vi "MGCC_PVFcst_main.vi"() -> ()   [LabVIEW 2016]
doc: "-----------------------------------------------------------------------------------------------------------------------\nCopyright <2019> <The University of Tennessee at Knoxville and the University of Tennessee Research Foundation>\nThis software is released under BSD-3 \nhttps://opensource.org/licenses/BSD-3-Clause \nAdditional license options available at https://utrf.tennessee.edu/industry/sample-agreements/\n-----------------------------------------------------------------------------------------------------------------------\n\n\nThis VI implements a PV forecasting algorithm using ARMA regression. The measurements from the PV local controller are taken every 15 minutes, and are stored using shared variables. Weather information is assumed to be available, and is transmitted through communication. The VI distinguishes between sunny and overcast days, but more detailed classification of cloud cover can be achieved using the same approach (case structure). The VI calls Sub-VI \"MGCC_PVFcst_PF.vi\" to train and generate forecasts for the next 24-hour period. If an alternative timing source is available, the timers in this VI can be replaced for free control of the triggering of this VI."
uses:
  Sub-VIs/f_MGCC_PVFcst_ActualPV.vi
  Finite State Machine/Sub-VIs/MGCC_FntStaMach_gobal.vi
  Finite State Machine/Sub-VIs/MGCC_FntStaMach_PV_Mode.vi
  Communication/Global communication.vi
  Communication/Global communication output.vi
  <vilib>/Utility/error.llb/Error Cluster From Error Code.vi
  <vilib>/ErrorRing/Error Ring.xnode
  <vilib>/Analysis/NI_AALBase.lvlib
  Lib/MGCC_PVFcst_dataIO.lvlib
panel:
  out "f_MGCC_PVFcst_HistoricalPV_Overcast":dbl[](graph)
  out "Forecast_overcast":dbl[](graph)
  out "f_MGCC_PVFcst_HistoricalPV_Sunny":dbl[](graph)
  out "Forecast_sunny":dbl[](graph)
  out "error1":errorcluster
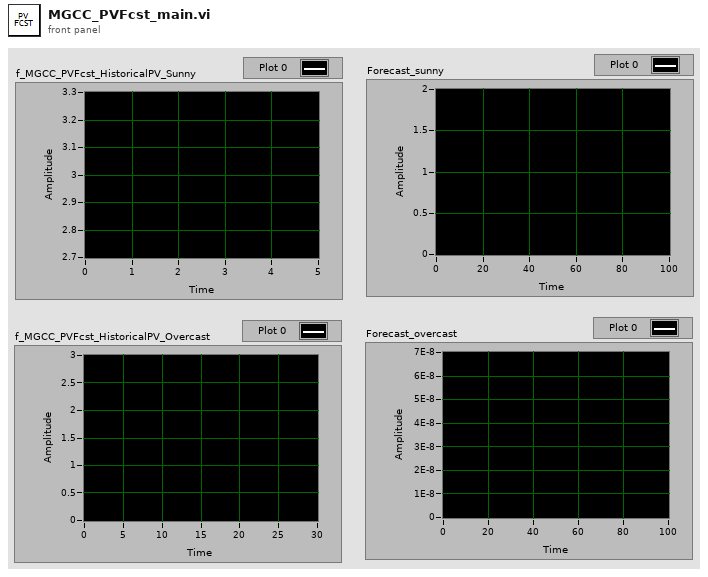
[diagram p1: front panel]
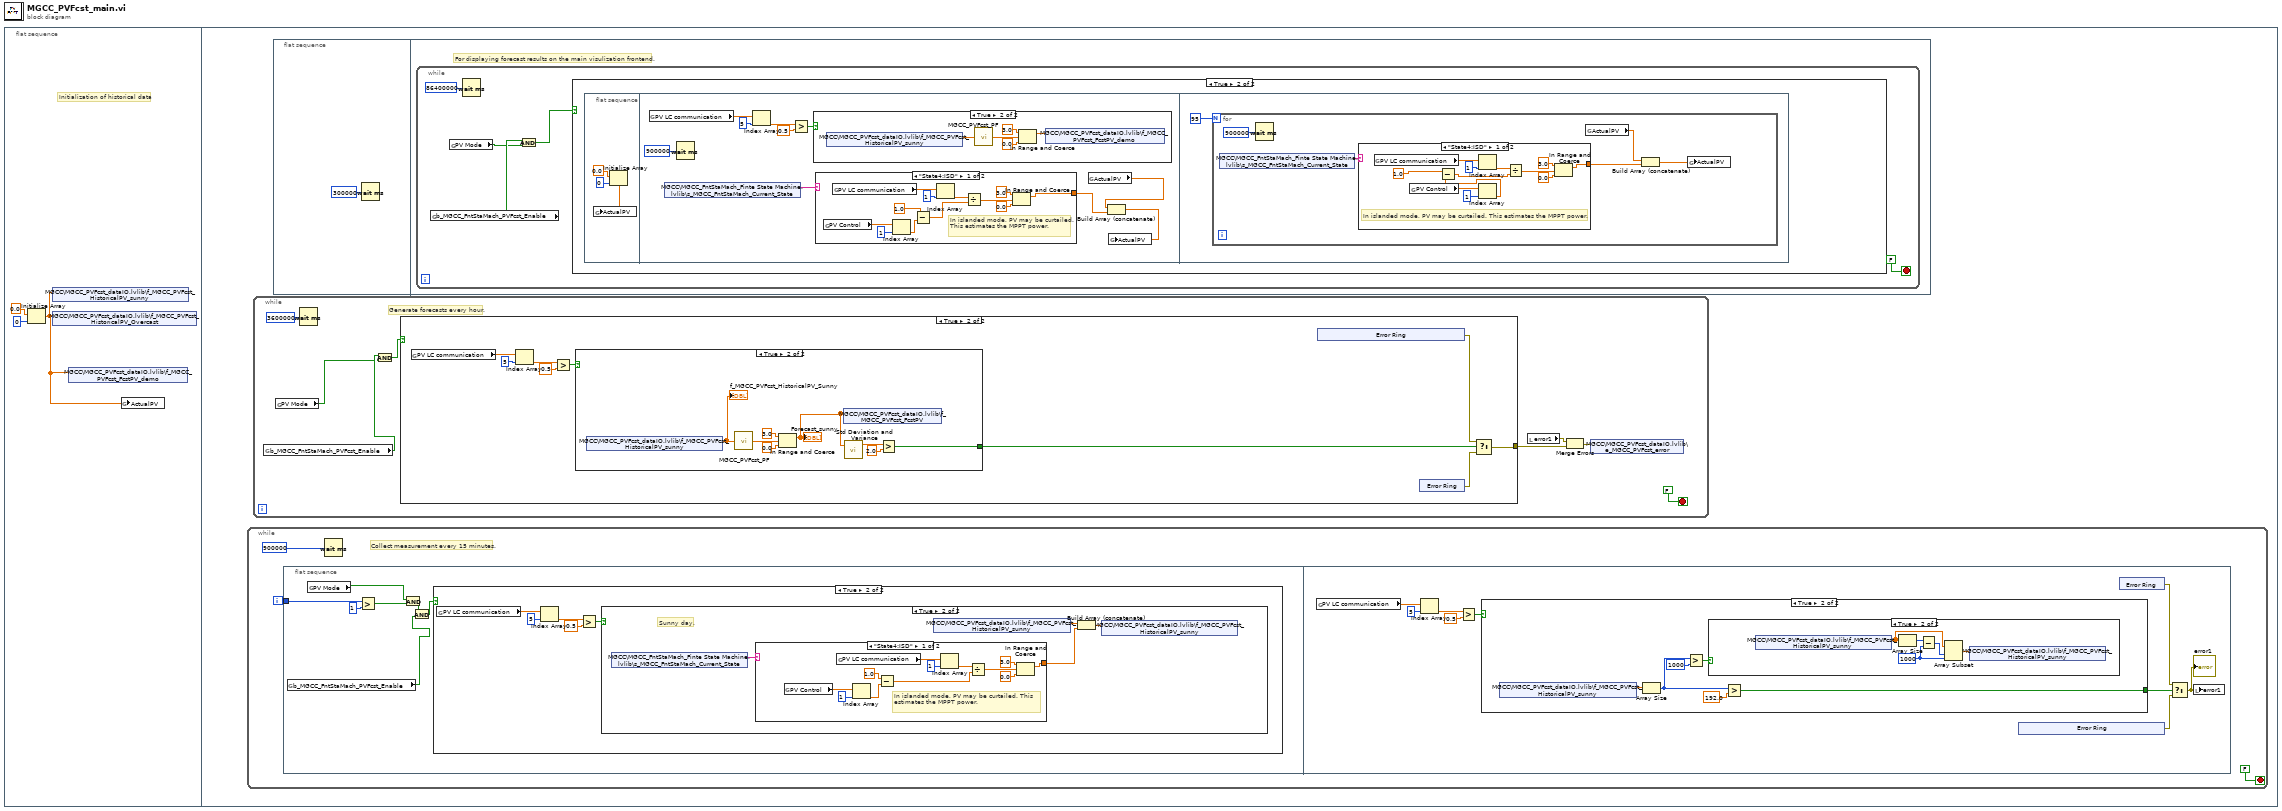
[diagram p0: block diagram]
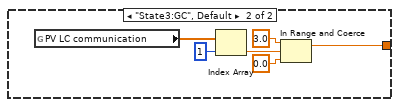
[diagram p3: hidden frame]
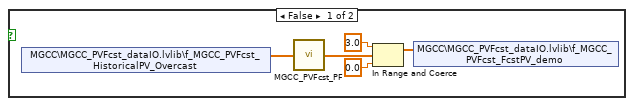
[diagram p4: hidden frame]
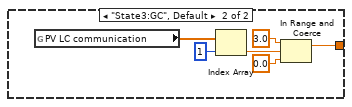
[diagram p5: hidden frame]
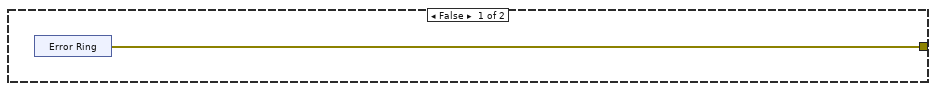
[diagram p6: hidden frame]
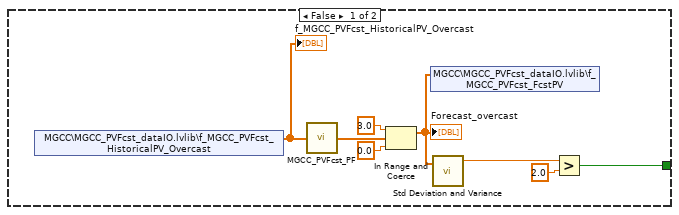
[diagram p7: hidden frame]
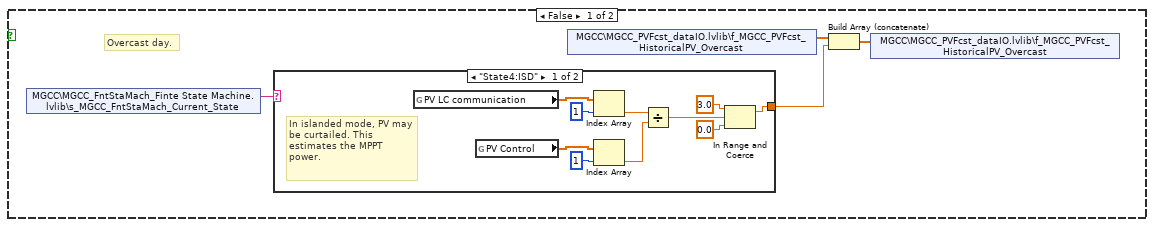
[diagram p9: hidden frame]
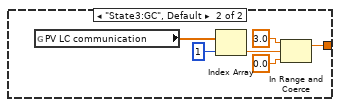
[diagram p10: hidden frame]
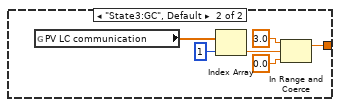
[diagram p11: hidden frame]
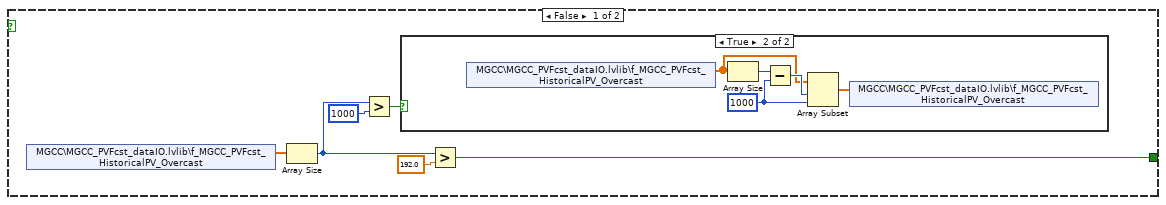
[diagram p12: hidden frame]
diagram:
  n1 = flat-sequence {
    frame #0 {
      # "Initialization of historical data"
      n2 = Initialize Array(0.0 ("element"), 0 ("dimension size")) -> (w1:dbl[])
      n3 = shared-variable "MGCC\\MGCC_PVFcst_dataIO.lvlib\\f_MGCC_PVFcst_HistoricalPV_sunny"(w1) -> ()  [unwired: 1 in, 1 out]
      n4 = shared-variable "MGCC\\MGCC_PVFcst_dataIO.lvlib\\f_MGCC_PVFcst_HistoricalPV_Overcast"(w1) -> ()  [unwired: 1 in, 1 out]
      n5 = shared-variable "MGCC\\MGCC_PVFcst_dataIO.lvlib\\f_MGCC_PVFcst_FcstPV_demo"(w1) -> ()  [unwired: 1 in, 1 out]
      n6 = global write "f_MGCC_PVFcst_ActualPV.vi" "ActualPV"(w1) -> ()
    }
    frame #1 {
      n7 = while {
        i -> [w116]
        stop <- FALSE stop-if-true
        # "Collect measurement every 15 minutes."
        n8 = flat-sequence {
          tunnel: w116 -> [w123]
          frame #0 {
            n9 = global read "MGCC_FntStaMach_gobal.vi" "b_MGCC_FntStaMach_PVFcst_Enable"() -> (w120:bool)
            n10 = global read "MGCC_FntStaMach_PV_Mode.vi" "PV Mode"() -> (w119:bool)
            n11 = Greater?(x=w123, y=1) -> (0:w124:bool)
            n12 = And(x=w119, y=w124) -> (x .and. y?=w122:bool)
            n13 = And(x=w122, y=w120) -> (x .and. y?=w121:bool)
            n14 = case shown="True" w121 {
              frame False {
              }
              frame True {
                n15 = global read "Global communication.vi" "PV LC communication"() -> (w130:dbl[])
                n16 = Index Array(array=w130, index=5) -> (element=w128:dbl)
                n17 = Greater?(x=w128, y=0.5) -> (0:w126:bool)
                n18 = case shown="True" w126 {
                  frame False {
                    # "Overcast day."
                    n19 = shared-variable "MGCC\\MGCC_FntStaMach_Finte State Machine.lvlib\\s_MGCC_FntStaMach_Current_State"() -> (w131:string)  [unwired: 1 in, 1 out]
                    n20 = case shown="\"State4:ISD\"" w131 {
                      tunnel: [w135 w148] -> w132
                      frame "State4:ISD" {
                        # "In islanded mode, PV may be curtailed. This estimates the MPPT power."
                        n21 = global read "Global communication.vi" "PV LC communication"() -> (w142:dbl[])
                        n22 = global read "Global communication output.vi" "PV Control"() -> (w139:dbl[])
                        n23 = Index Array(array=w142, index=1) -> (element=w136:dbl)
                        n24 = Index Array(array=w139, index=1) -> (element=w138:dbl)
                        n25 = Divide(x=w136, y=w138) -> (x/y=w137:dbl)
                        n26 = In Range and Coerce(upper limit=3.0, x=w137, lower limit=0.0) -> (coerced(x)=w135:dbl)  [unwired: 1 out]
                      }
                      frame "State3:GC", Default {
                        n27 = global read "Global communication.vi" "PV LC communication"() -> (w147:dbl[])
                        n28 = Index Array(array=w147, index=1) -> (element=w145:dbl)
                        n29 = In Range and Coerce(upper limit=3.0, x=w145, lower limit=0.0) -> (coerced(x)=w148:dbl)  [unwired: 1 out]
                      }
                    }
                    n30 = shared-variable "MGCC\\MGCC_PVFcst_dataIO.lvlib\\f_MGCC_PVFcst_HistoricalPV_Overcast"() -> (w134:dbl[])  [unwired: 1 in, 1 out]
                    n31 = Build Array (concatenate)(w134, w132) -> (w133:dbl[])
                    n32 = shared-variable "MGCC\\MGCC_PVFcst_dataIO.lvlib\\f_MGCC_PVFcst_HistoricalPV_Overcast"(w133) -> ()  [unwired: 1 in, 1 out]
                  }
                  frame True {
                    # "Sunny day."
                    n33 = shared-variable "MGCC\\MGCC_FntStaMach_Finte State Machine.lvlib\\s_MGCC_FntStaMach_Current_State"() -> (w152:string)  [unwired: 1 in, 1 out]
                    n34 = case shown="\"State4:ISD\"" w152 {
                      tunnel: [w158 w170] -> w151
                      frame "State4:ISD" {
                        # "In islanded mode, PV may be curtailed. This estimates the MPPT power."
                        n35 = global read "Global communication output.vi" "PV Control"() -> (w161:dbl[])
                        n36 = global read "Global communication.vi" "PV LC communication"() -> (w164:dbl[])
                        n37 = Index Array(array=w161, index=1) -> (element=w157:dbl)
                        n38 = Subtract(x=1.0, y=w157) -> (x-y=w155:dbl)
                        n39 = Index Array(array=w164, index=1) -> (element=w159:dbl)
                        n40 = Divide(x=w159, y=w155) -> (x/y=w160:dbl)
                        n41 = In Range and Coerce(upper limit=3.0, x=w160, lower limit=0.0) -> (coerced(x)=w158:dbl)  [unwired: 1 out]
                      }
                      frame "State3:GC", Default {
                        n42 = global read "Global communication.vi" "PV LC communication"() -> (w169:dbl[])
                        n43 = Index Array(array=w169, index=1) -> (element=w167:dbl)
                        n44 = In Range and Coerce(upper limit=3.0, x=w167, lower limit=0.0) -> (coerced(x)=w170:dbl)  [unwired: 1 out]
                      }
                    }
                    n45 = shared-variable "MGCC\\MGCC_PVFcst_dataIO.lvlib\\f_MGCC_PVFcst_HistoricalPV_sunny"() -> (w154:dbl[])  [unwired: 1 in, 1 out]
                    n46 = Build Array (concatenate)(w154, w151) -> (w153:dbl[])
                    n47 = shared-variable "MGCC\\MGCC_PVFcst_dataIO.lvlib\\f_MGCC_PVFcst_HistoricalPV_sunny"(w153) -> ()  [unwired: 1 in, 1 out]
                  }
                }
              }
            }
          }
          frame #1 {
            n48 = global read "Global communication.vi" "PV LC communication"() -> (w177:dbl[])
            n49 = Index Array(array=w177, index=5) -> (element=w175:dbl)
            n50 = Greater?(x=w175, y=0.5) -> (0:w173:bool)
            n51 = case shown="True" w173 {
              tunnel: [w183 w193] -> w179
              frame False {
                n52 = shared-variable "MGCC\\MGCC_PVFcst_dataIO.lvlib\\f_MGCC_PVFcst_HistoricalPV_Overcast"() -> (w184:dbl[])  [unwired: 1 in, 1 out]
                n53 = Array Size(array=w184) -> (size(s)=w187:i32)
                n54 = Greater?(x=w187, y=1000) -> (0:w182:bool)
                n55 = case shown="True" w182 {
                  frame False {
                  }
                  frame True {
                    w192 = 1000 ("y")
                    n56 = shared-variable "MGCC\\MGCC_PVFcst_dataIO.lvlib\\f_MGCC_PVFcst_HistoricalPV_Overcast"() -> (w188:dbl[])  [unwired: 1 in, 1 out]
                    n57 = Array Size(array=w188) -> (size(s)=w189:i32)
                    n58 = Subtract(x=w189, y=w192) -> (x-y=w190:i32)
                    n59 = Array Subset(array=w188, index=w190, length=w192) -> (w191:dbl[])
                    n60 = shared-variable "MGCC\\MGCC_PVFcst_dataIO.lvlib\\f_MGCC_PVFcst_HistoricalPV_Overcast"(w191) -> ()  [unwired: 1 in, 1 out]
                  }
                }
                n61 = Greater?(x=w187, y=192.0) -> (0:w183:bool)
              }
              frame True {
                n62 = shared-variable "MGCC\\MGCC_PVFcst_dataIO.lvlib\\f_MGCC_PVFcst_HistoricalPV_sunny"() -> (w198:dbl[])  [unwired: 1 in, 1 out]
                n63 = Array Size(array=w198) -> (size(s)=w194:i32)
                n64 = Greater?(x=w194, y=1000) -> (0:w196:bool)
                n65 = case shown="True" w196 {
                  frame False {
                  }
                  frame True {
                    w199 = 1000 ("y")
                    n66 = shared-variable "MGCC\\MGCC_PVFcst_dataIO.lvlib\\f_MGCC_PVFcst_HistoricalPV_sunny"() -> (w203:dbl[])  [unwired: 1 in, 1 out]
                    n67 = Array Size(array=w203) -> (size(s)=w202:i32)
                    n68 = Subtract(x=w202, y=w199) -> (x-y=w201:i32)
                    n69 = Array Subset(array=w203, index=w201, length=w199) -> (w200:dbl[])
                    n70 = shared-variable "MGCC\\MGCC_PVFcst_dataIO.lvlib\\f_MGCC_PVFcst_HistoricalPV_sunny"(w200) -> ()  [unwired: 1 in, 1 out]
                  }
                }
                n71 = Greater?(x=w194, y=192.0) -> (0:w193:bool)
              }
            }
            n72 = xnode "Error Ring"() -> ("error out"=w180:errorcluster)
            n73 = xnode "Error Ring"() -> ("error out"=w181:errorcluster)
            n74 = Select(t=w181, s=w179, f=w180) -> (s? t:f=w178:errorcluster)
            "error1" <- w178
            n75 = local write "error1"(w178) -> ()
          }
        }
        n76 = Wait (ms)(milliseconds to wait=u32 900000) -> ()  [unwired: 1 out]
      }
      n77 = while {
        stop <- FALSE stop-if-true
        # "Generate forecasts every hour."
        n78 = global read "MGCC_FntStaMach_gobal.vi" "b_MGCC_FntStaMach_PVFcst_Enable"() -> (w76:bool)
        n79 = global read "MGCC_FntStaMach_PV_Mode.vi" "PV Mode"() -> (w75:bool)
        n80 = Wait (ms)(milliseconds to wait=u32 3600000) -> ()  [unwired: 1 out]
        n81 = And(x=w76, y=w75) -> (x .and. y?=w77:bool)
        n82 = case shown="True" w77 {
          tunnel: [w83 w90] -> w80
          frame False {
            n83 = xnode "Error Ring"() -> ("error out"=w83:errorcluster)
          }
          frame True {
            n84 = global read "Global communication.vi" "PV LC communication"() -> (w89:dbl[])
            n85 = Index Array(array=w89, index=5) -> (element=w87:dbl)
            n86 = Greater?(x=w87, y=0.5) -> (0:w85:bool)
            n87 = case shown="True" w85 {
              tunnel: [w94 w102] -> w91
              frame False {
                n88 = shared-variable "MGCC\\MGCC_PVFcst_dataIO.lvlib\\f_MGCC_PVFcst_HistoricalPV_Overcast"() -> (w95:dbl[])  [unwired: 1 in, 1 out]
                "f_MGCC_PVFcst_HistoricalPV_Overcast" <- w95
                n89 = call "MGCC_PVFcst_PF.vi"("InputTimeSeries"=w95) -> ("predicted series"=w98:dbl[])
                n90 = In Range and Coerce(upper limit=3.0, x=w98, lower limit=0.0) -> (coerced(x)=w101:dbl[])  [unwired: 1 out]
                "Forecast_overcast" <- w101
                n91 = shared-variable "MGCC\\MGCC_PVFcst_dataIO.lvlib\\f_MGCC_PVFcst_FcstPV"(w101) -> ()  [unwired: 1 in, 1 out]
                n92 = call <vilib>:"Std Deviation and Variance.vi"("X"=w101) -> ("mean"=w100:dbl)  [unwired: 1 in, 2 out]
                n93 = Greater?(x=w100, y=2.0) -> (0:w94:bool)
              }
              frame True {
                n94 = shared-variable "MGCC\\MGCC_PVFcst_dataIO.lvlib\\f_MGCC_PVFcst_HistoricalPV_sunny"() -> (w109:dbl[])  [unwired: 1 in, 1 out]
                "f_MGCC_PVFcst_HistoricalPV_Sunny" <- w109
                n95 = call "MGCC_PVFcst_PF.vi"("InputTimeSeries"=w109) -> ("predicted series"=w106:dbl[])
                n96 = In Range and Coerce(upper limit=3.0, x=w106, lower limit=0.0) -> (coerced(x)=w103:dbl[])  [unwired: 1 out]
                "Forecast_sunny" <- w103
                n97 = shared-variable "MGCC\\MGCC_PVFcst_dataIO.lvlib\\f_MGCC_PVFcst_FcstPV"(w103) -> ()  [unwired: 1 in, 1 out]
                n98 = call <vilib>:"Std Deviation and Variance.vi"("X"=w103) -> ("mean"=w104:dbl)  [unwired: 1 in, 2 out]
                n99 = Greater?(x=w104, y=2.0) -> (0:w102:bool)
              }
            }
            n100 = xnode "Error Ring"() -> ("error out"=w93:errorcluster)
            n101 = xnode "Error Ring"() -> ("error out"=w92:errorcluster)
            n102 = Select(t=w93, s=w91, f=w92) -> (s? t:f=w90:errorcluster)
          }
        }
        n103 = local read "error1"() -> (w78:errorcluster)
        n104 = Merge Errors(w78, w80) -> (w79:errorcluster)
        n105 = shared-variable "MGCC\\MGCC_PVFcst_dataIO.lvlib\\e_MGCC_PVFcst_error"(w79) -> ()  [unwired: 1 in, 1 out]
      }
      n106 = flat-sequence {
        frame #0 {
          n107 = Wait (ms)(milliseconds to wait=u32 300000) -> ()  [unwired: 1 out]
        }
        frame #1 {
          # "For displaying forecast results on the main visulization frontend."
          n108 = while {
            stop <- FALSE stop-if-true
            n109 = global read "MGCC_FntStaMach_gobal.vi" "b_MGCC_FntStaMach_PVFcst_Enable"() -> (w6:bool)
            n110 = global read "MGCC_FntStaMach_PV_Mode.vi" "PV Mode"() -> (w5:bool)
            n111 = Wait (ms)(milliseconds to wait=u32 86400000) -> ()  [unwired: 1 out]
            n112 = And(x=w6, y=w5) -> (x .and. y?=w7:bool)
            n113 = case shown="True" w7 {
              frame False {
              }
              frame True {
                n114 = flat-sequence {
                  frame #0 {
                    n115 = Initialize Array(0.0 ("element"), 0 ("dimension size")) -> (w12:dbl[])
                    n116 = global write "f_MGCC_PVFcst_ActualPV.vi" "ActualPV"(w12) -> ()
                  }
                  frame #1 {
                    n117 = global read "Global communication.vi" "PV LC communication"() -> (w22:dbl[])
                    n118 = shared-variable "MGCC\\MGCC_FntStaMach_Finte State Machine.lvlib\\s_MGCC_FntStaMach_Current_State"() -> (w17:string)  [unwired: 1 in, 1 out]
                    n119 = Wait (ms)(milliseconds to wait=u32 900000) -> ()  [unwired: 1 out]
                    n120 = Index Array(array=w22, index=5) -> (element=w20:dbl)
                    n121 = Greater?(x=w20, y=0.5) -> (0:w18:bool)
                    n122 = case shown="True" w18 {
                      frame False {
                        n123 = shared-variable "MGCC\\MGCC_PVFcst_dataIO.lvlib\\f_MGCC_PVFcst_HistoricalPV_Overcast"() -> (w41:dbl[])  [unwired: 1 in, 1 out]
                        n124 = call "MGCC_PVFcst_PF.vi"("InputTimeSeries"=w41) -> ("predicted series"=w44:dbl[])
                        n125 = In Range and Coerce(upper limit=3.0, x=w44, lower limit=0.0) -> (coerced(x)=w45:dbl[])  [unwired: 1 out]
                        n126 = shared-variable "MGCC\\MGCC_PVFcst_dataIO.lvlib\\f_MGCC_PVFcst_FcstPV_demo"(w45) -> ()  [unwired: 1 in, 1 out]
                      }
                      frame True {
                        n127 = shared-variable "MGCC\\MGCC_PVFcst_dataIO.lvlib\\f_MGCC_PVFcst_HistoricalPV_sunny"() -> (w50:dbl[])  [unwired: 1 in, 1 out]
                        n128 = call "MGCC_PVFcst_PF.vi"("InputTimeSeries"=w50) -> ("predicted series"=w47:dbl[])
                        n129 = In Range and Coerce(upper limit=3.0, x=w47, lower limit=0.0) -> (coerced(x)=w46:dbl[])  [unwired: 1 out]
                        n130 = shared-variable "MGCC\\MGCC_PVFcst_dataIO.lvlib\\f_MGCC_PVFcst_FcstPV_demo"(w46) -> ()  [unwired: 1 in, 1 out]
                      }
                    }
                    n131 = case shown="\"State4:ISD\"" w17 {
                      tunnel: [w26 w38] -> w15
                      frame "State4:ISD" {
                        # "In islanded mode, PV may be curtailed. This estimates the MPPT power."
                        n132 = global read "Global communication output.vi" "PV Control"() -> (w29:dbl[])
                        n133 = global read "Global communication.vi" "PV LC communication"() -> (w32:dbl[])
                        n134 = Index Array(array=w29, index=1) -> (element=w25:dbl)
                        n135 = Subtract(x=1.0, y=w25) -> (x-y=w23:dbl)
                        n136 = Index Array(array=w32, index=1) -> (element=w27:dbl)
                        n137 = Divide(x=w27, y=w23) -> (x/y=w28:dbl)
                        n138 = In Range and Coerce(upper limit=3.0, x=w28, lower limit=0.0) -> (coerced(x)=w26:dbl)  [unwired: 1 out]
                      }
                      frame "State3:GC", Default {
                        n139 = global read "Global communication.vi" "PV LC communication"() -> (w37:dbl[])
                        n140 = Index Array(array=w37, index=1) -> (element=w35:dbl)
                        n141 = In Range and Coerce(upper limit=3.0, x=w35, lower limit=0.0) -> (coerced(x)=w38:dbl)  [unwired: 1 out]
                      }
                    }
                    n142 = global read "f_MGCC_PVFcst_ActualPV.vi" "ActualPV"() -> (w14:dbl[])
                    n143 = Build Array (concatenate)(w14, w15) -> (w13:dbl[])
                    n144 = global write "f_MGCC_PVFcst_ActualPV.vi" "ActualPV"(w13) -> ()
                  }
                  frame #2 {
                    n145 = for {
                      N: 95 -> [_]
                      n146 = shared-variable "MGCC\\MGCC_FntStaMach_Finte State Machine.lvlib\\s_MGCC_FntStaMach_Current_State"() -> (w55:string)  [unwired: 1 in, 1 out]
                      n147 = Wait (ms)(milliseconds to wait=u32 900000) -> ()  [unwired: 1 out]
                      n148 = case shown="\"State4:ISD\"" w55 {
                        tunnel: [w60 w72] -> w54
                        frame "State4:ISD" {
                          # "In islanded mode, PV may be curtailed. This estimates the MPPT power."
                          n149 = global read "Global communication.vi" "PV LC communication"() -> (w66:dbl[])
                          n150 = global read "Global communication output.vi" "PV Control"() -> (w63:dbl[])
                          n151 = Index Array(array=w66, index=1) -> (element=w61:dbl)
                          n152 = Index Array(array=w63, index=1) -> (element=w58:dbl)
                          n153 = Subtract(x=1.0, y=w58) -> (x-y=w57:dbl)
                          n154 = Divide(x=w61, y=w57) -> (x/y=w62:dbl)
                          n155 = In Range and Coerce(upper limit=3.0, x=w62, lower limit=0.0) -> (coerced(x)=w60:dbl)  [unwired: 1 out]
                        }
                        frame "State3:GC", Default {
                          n156 = global read "Global communication.vi" "PV LC communication"() -> (w71:dbl[])
                          n157 = Index Array(array=w71, index=1) -> (element=w69:dbl)
                          n158 = In Range and Coerce(upper limit=3.0, x=w69, lower limit=0.0) -> (coerced(x)=w72:dbl)  [unwired: 1 out]
                        }
                      }
                      n159 = global read "f_MGCC_PVFcst_ActualPV.vi" "ActualPV"() -> (w52:dbl[])
                      n160 = Build Array (concatenate)(w52, w54) -> (w53:dbl[])
                      n161 = global write "f_MGCC_PVFcst_ActualPV.vi" "ActualPV"(w53) -> ()
                    }
                  }
                }
              }
            }
          }
        }
      }
    }
  }
